vi "array -- bilinear regression 2D -- curvature wrapper -- V1.vi"(7 "action":T6, 8 "2D curvature tensor IN":T1={"curvature Matrix"=[[3.0, 1.0], [1.0, 4.0]], "eigenvs"=[4.618033988749895, 2.381966011250105], "Eigenvectors"=[[-0.8506508083520399+0.0i, -0.5257311121191335+0.0i], [0.5257311121191335+0.0i, -0.8506508083520399+0.0i]], "theta (rad)"=0.5535743588970453, "theta (deg)"=31.717474411461012, "Δs"=[4.618033988749895, 2.381966011250105], "δG/G"=0.5535743588970453, "δs"=[4.618033988749895, 2.381966011250105], "inverse Matrix"=[[3.0, 1.0], [1.0, 4.0]], "noise T"=0.5535743588970453, "pars & errors"={}} {"noise T" format="%#_3p"; "inverse Matrix" format="%#_3p"; "δs" format="%#_2p"; "δG/G" format="%#_3p"; "Δs" format="%#_3p"; "theta (deg)" format="%#_3p"; "curvature Matrix" format="%#_3p"; "eigenvs" format="%#_3p"; "Eigenvectors" format="%#_3p"; "theta (rad)" format="%#_3p"}, 10 "fit  IN":dbl[](array[numeric])=[1.9, 2.6, 3.3, 1.0, 2.7, 3.9], 11 "xyz IN":cluster{"x":dbl[], "y":dbl[], "z":dbl[]}={"x"=[10.0, -7.0, 6.0, -1.0, -1.0, -1.0, 1.0, 1.0], "y"=[-1.0, 4.0, 45.0, -1.0, -23.0, 1.0, -1.0, 2.0], "z"=[1.0, -5.0, 1.0, 4.0, 1.0, 43.0, -4.0, 12.0]}) -> (0 "2D curvature tensor OUT":T1={"curvature Matrix"=[[0.9999999999999996, 0.9999999999999998], [0.9999999999999998, 1.0]], "eigenvs"=[1.7838428397948585, 0.21615716020514097], "Eigenvectors"=[[-0.8506508083520399+0.0i, -0.5257311121191335+0.0i], [0.5257311121191335+0.0i, -0.8506508083520399+0.0i]], "theta (rad)"=0.7853981633974482, "theta (deg)"=44.99999999999999, "Δs"=[nan, nan], "δG/G"=0.5535743588970453, "δs"=[4.618033988749895, 2.381966011250105], "inverse Matrix"=[], "noise T"=0.5535743588970453, "pars & errors"={}} {"noise T" format="%#_3p"; "inverse Matrix" format="%#_3p"; "δs" format="%#_2p"; "δG/G" format="%#_3p"; "Δs" format="%#_3p"; "theta (deg)" format="%#_3p"; "curvature Matrix" format="%#_3p"; "eigenvs" format="%#_3p"; "Eigenvectors" format="%#_3p"; "theta (rad)" format="%#_3p"}, 1 "fit map out":map{T5, dbl}(c390)={enum."1"=0.0, enum."x"=0.0, enum."y"=1.1102230246251565e-16, enum."xx"=0.9999999999999996, enum."xy"=0.9999999999999998, enum."yy"=1.0}, 2 "fit OUT":dbl[](array[numeric])=[0.9999999999999996, 0.9999999999999998, 1.0, 0.0, 1.1102230246251565e-16, 0.0], 3 "xyz OUT":cluster{"x":dbl[], "y":dbl[], "z":dbl[]}={"x"=[0.0, 0.0, 0.0, -1.0, -1.0, -1.0, 1.0, 1.0], "y"=[-1.0, 0.0, 1.0, -1.0, 0.0, 1.0, -1.0, 0.0], "z"=[1.0, 0.0, 1.0, 4.0, 1.0, 0.0, 0.0, 1.0]})   [LabVIEW 2021]
uses:
  array -- fit control .ctl
  array -- bilinear regression 2D.ctl
  <vilib>/Analysis/Matrix/Datatypes/RealMatrix.ctl
  2D curvature tensor.ctl
  <vilib>/Analysis/Matrix/Datatypes/ComplexMatrix.ctl
  3-lorentzian-parameters.ctl
  2D curvature tensor actions.ctl
  <vilib>/Analysis/baseanly.llb/A x B.vi
  <vilib>/Analysis/baseanly.llb/Real A x B.vi
  <vilib>/Analysis/Matrix/Numeric/Conversions/Array To Matrix - RA2.vi
  <vilib>/Analysis/baseanly.llb/Inverse Matrix.vi
  <vilib>/Analysis/baseanly.llb/Real Inverse Matrix.vi
  <vilib>/Analysis/Matrix/Numeric/Conversions/Matrix To Array.vi
  <vilib>/Analysis/Matrix/Numeric/Conversions/Matrix To Array - RM.vi
  <vilib>/Analysis/Matrix/NI_Matrix.lvlib
panel:
  out "curvature Matrix":T2=[[0.9999999999999996, 0.9999999999999998], [0.9999999999999998, 1.0]]
  out "y OUT":dbl[](array[numeric])=[-1.0, 0.0, 1.0, -1.0, 0.0, 1.0, -1.0, 0.0]
  out "y":dbl[](array[numeric])=[-1.0, 0.0, 1.0, -1.0, 0.0, 1.0, -1.0, 0.0]
  out "x OUT":dbl[](array[numeric])=[0.0, 0.0, 0.0, -1.0, -1.0, -1.0, 1.0, 1.0]
  out "z OUT":dbl[](array[numeric])=[1.0, 0.0, 1.0, 4.0, 1.0, 0.0, 0.0, 1.0]
  out "z":dbl[](array[numeric])=[1.0, 0.0, 1.0, 4.0, 1.0, 0.0, 0.0, 1.0]
  out "x":dbl[](array[numeric])=[0.0, 0.0, 0.0, -1.0, -1.0, -1.0, 1.0, 1.0]
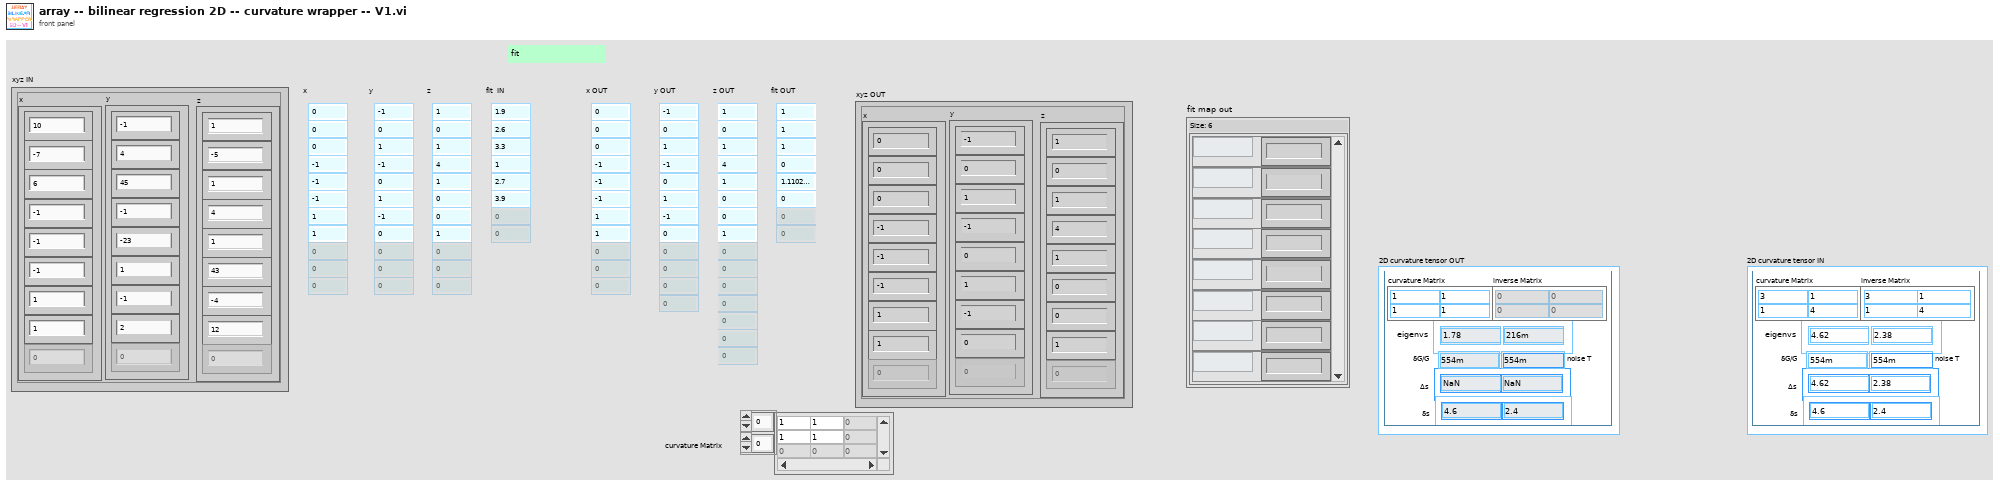
[diagram p1: front panel]
types:
  T1 = typedef "2D curvature tensor.ctl" = cluster{"curvature Matrix":T2, "eigenvs":dbl[], "Eigenvectors":T3, "theta (rad)":dbl, "theta (deg)":dbl, "Δs":dbl[], "δG/G":dbl, "δs":dbl[], "inverse Matrix":T2, "noise T":dbl, "pars & errors":map{T4, dbl}}
  T2 = typedef "NI_Matrix.lvlib/RealMatrix.ctl" = dbl[][]
  T3 = typedef "NI_Matrix.lvlib/ComplexMatrix.ctl" = cdb[][]
  T4 = typedef "3-lorentzian-parameters.ctl" = enum16{"ζ", "τ1", "τS", "τN", "τC", "κ0", "m1", "m2", "m3", "T (K)", "B (T)", "θ (deg)", "side (S|R)", "set of (B|T)", "Re(offset)", "Im(offset)", "στ1", "στ1-", "στ1+", "στS", "στS-", "στS+", "στN", "στN-", "στN+"}
  T5 = typedef "array -- bilinear regression 2D.ctl" = enum16{"1", "x", "y", "xx", "xy", "yy", "xxy", "xyy", "yyy", "xxx", "xxyy", "xyyy", "xxxy", "yyyy", "xxxx", "xxz", "xyz", "yyz", "xz", "yz", "z"}
  T6 = typedef "array -- fit control .ctl" = enum16{"fit", "calc", "check", "init"}
  T7 = typedef "2D curvature tensor actions.ctl" = enum16{"eigensystem", "sigma", "set matrix", "inverse"}
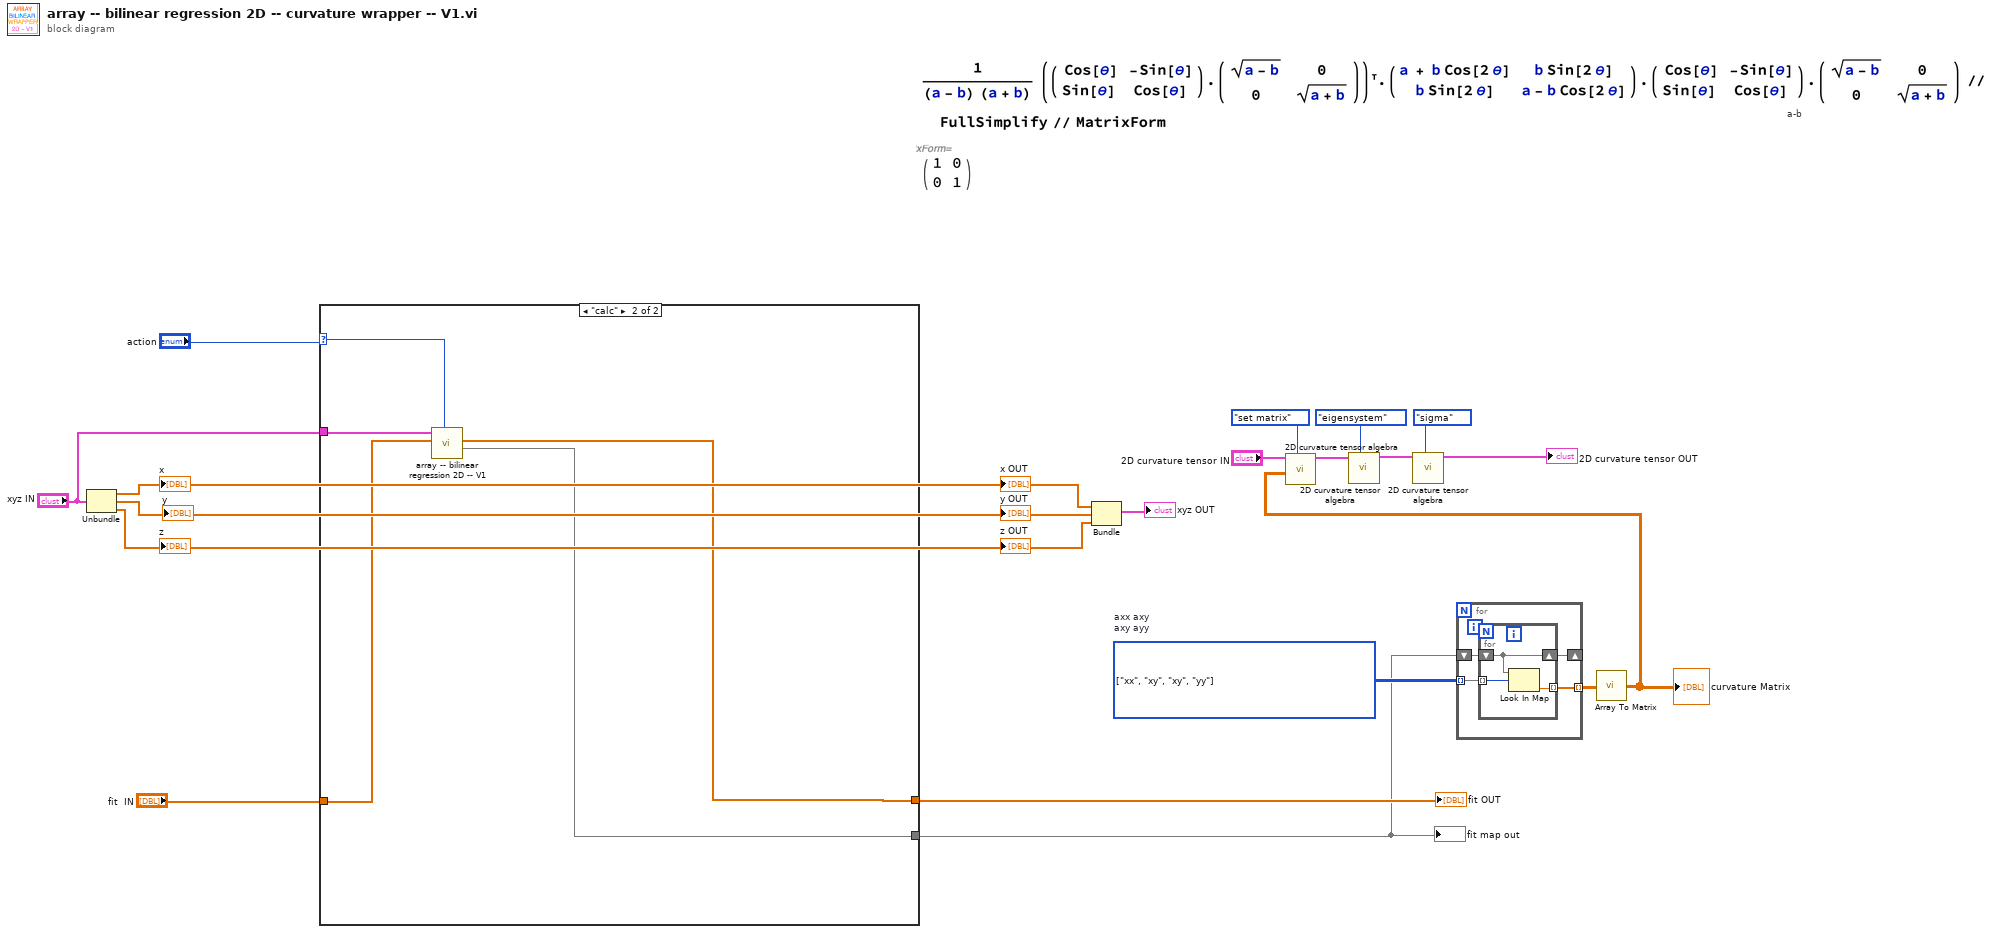
[diagram p0: block diagram]
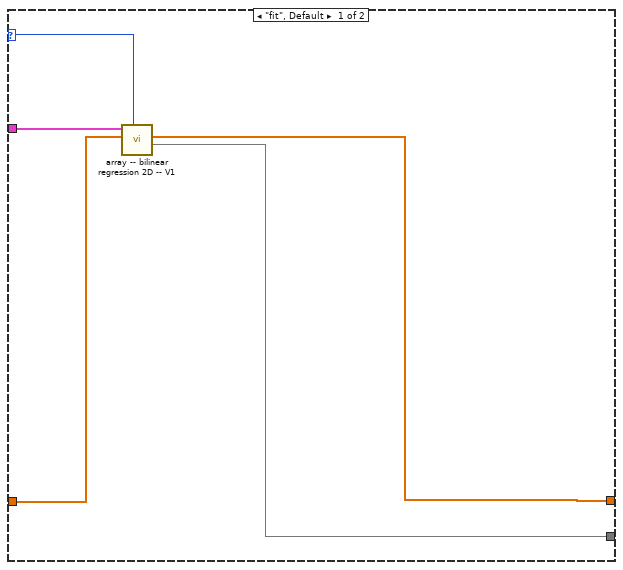
[diagram p2: hidden frame]
diagram:
  w17 = T5[][] [[enum."xx", enum."xy"], [enum."xy", enum."yy"]] items=["1", "x", "y", "xx", "xy", "yy", "xxy", "xyy", "yyy", "xxx", "xxyy", "xyyy", "xxxy", "yyyy", "xxxx", "xxz", "xyz", "yyz", "xz", "yz", "z"]  # axx axy axy ayy
  # "a-b"
  n1 = Unbundle("xyz IN") -> ("x"=w8:dbl[], "y"=w7:dbl[], "z"=w6:dbl[])
  "x" <- w8
  "z" <- w6
  "z OUT" <- w6
  "x OUT" <- w8
  "y OUT" <- w7
  "y" <- w7
  n2 = case shown="\"calc\"" "action" {
    selector: "action" -> [w21 w26]
    tunnel: "xyz IN" -> [w24 w29]
    tunnel: [w23 w28] -> w4
    tunnel: [w22 w27] -> w3
    tunnel: "fit  IN" -> [w20 w25]
    frame "fit", Default {
      n3 = call "array -- bilinear regression 2D -- V1.vi"("action"=w21, "fit  IN"=w20, "xyz IN"=w24) -> ("fit map out"=w22:map{T5, dbl}, "fit OUT"=w23:dbl[])  [unwired: 6 in, 1 out]
    }
    frame "calc" {
      n4 = call "array -- bilinear regression 2D -- V1.vi"("action"=w26, "fit  IN"=w25, "xyz IN"=w29) -> ("fit map out"=w27:map{T5, dbl}, "fit OUT"=w28:dbl[])  [unwired: 6 in, 1 out]
    }
  }
  "fit OUT" <- w4
  "fit map out" <- w3
  n5 = Bundle("x"=w8, "y"=w7, "z"=w6) -> (→"xyz OUT":cluster{"x":dbl[], "y":dbl[], "z":dbl[]})  [unwired: 1 in]
  n6 = for {
    tunnel: w17 -> [w33] mode=indexing
    shift-right: [w31] -> _
    shift-left: w3 -> [w32]
    tunnel: [w30] -> w18 mode=indexing
    n7 = for {
      tunnel: w33 -> [w35] mode=indexing
      shift-right: [w36] -> w31
      shift-left: w32 -> [w36]
      tunnel: [w34] -> w30 mode=indexing
      n8 = Look In Map(map=w36, key=w35) -> (value=w34:dbl)  [unwired: 1 in, 1 out]
    }
  }
  n9 = call-poly <vilib>:"Array To Matrix.vi"("Real 2D Array"=w18) -> ("Real Matrix"=w13:T2)
  "curvature Matrix" <- w13
  n10 = call "2D curvature tensor algebra.vi"("2D tensor"=2D_curvature_tensor_actions."set matrix", "2D curvature Matrix IN"=w13, "curvature tensor IN"="2D curvature tensor IN") -> ("curvature tensor OUT"=w15:T1)  [unwired: 7 in, 1 out]
  n11 = call "2D curvature tensor algebra.vi"("2D tensor"=2D_curvature_tensor_actions."eigensystem", "curvature tensor IN"=w15) -> ("curvature tensor OUT"=w12:T1)  [unwired: 8 in, 1 out]
  n12 = call "2D curvature tensor algebra.vi"("2D tensor"=2D_curvature_tensor_actions."sigma", "curvature tensor IN"=w12) -> ("curvature tensor OUT"=→"2D curvature tensor OUT":T1)  [unwired: 8 in, 1 out]
